vi "Name.vi"(11 "String Data Type in":refnum<class "String Data Type.lvclass">) -> (2 "String":string="Generic", 3 "String Data Type (dup)":refnum<class "String Data Type.lvclass">)   [LabVIEW 2018, in "String Data Type.lvclass"]
uses:
  String Data Type.lvclass
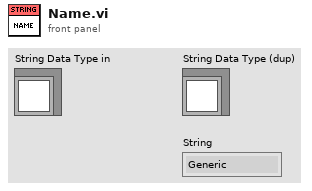
[diagram p1: front panel]
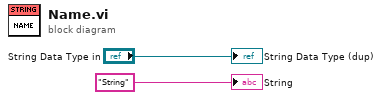
[diagram p0: block diagram]
diagram:
  "String Data Type (dup)" <- "String Data Type in"
  "String" <- "String" ("String")
